vi "GetAttributeViInt32_SA-Gating_Sweep.vi"(8 "error in (no error)":errorcluster {"code" format="%.0x"}, 9 "AttributeID":u32(ring)=1150537 items=["SA_GATING_DELAY_COMPENSATION"=1150537, "SA_GATING_METHOD"=1150529, "SA_GATING_SOURCE"=1150531, "SA_GATING_TYPE"=1150532, "SA_LISTSWEEP_ATTENUATION_ELECTRONIC_POINTS"=1150655, "SA_LISTSWEEP_ATTENUATION_MECHANICAL_POINTS"=1150656, "SA_LISTSWEEP_BANDWIDTH_RESOLUTION_POINTS"=1150634, "SA_LISTSWEEP_BANDWIDTH_RESOLUTION_TYPE_POINTS"=1150635, "SA_LISTSWEEP_BANDWIDTH_VIDEO_POINTS"=1150636, "SA_LISTSWEEP_DETECTOR_POINTS"=1150653, "SA_LISTSWEEP_FREQUENCY_POINTS"=1150638, "SA_LISTSWEEP_FREQUENCY_SYNTHESIS"=1150639, "SA_LISTSWEEP_SEQUENCE_POINTS"=1150643, "SA_LISTSWEEP_TIME_POINTS"=1150651, "SA_LISTSWEEP_TRIGGER_DELAY_POINTS"=1150645, "SA_LISTSWEEP_TRIGGER_HOLDOFF_POINTS"=1150646, "SA_LISTSWEEP_TRIGGER_LEVEL_POINTS"=1150647, "SA_LISTSWEEP_TRIGGER_SLOPE"=1150657, "SA_LISTSWEEP_TRIGGER_SLOPE_POINTS"=1150648, "SA_LISTSWEEP_TRIGGER_SOURCE_POINTS"=1150649, "SA_LISTSWEEP_TRIGGER_SOURCE"=1150658, "SA_SWEEPCOUPLING_BANDWIDTH_SHAPE"=1150730, "SA_SWEEPCOUPLING_BANDWIDTH_TYPE"=1150731, "SA_SWEEPCOUPLING_SWEEP_POINTS"=1150724, "SA_SWEEPCOUPLING_SWEEP_TIME_AUTO_RULES"=1150732, "SA_SWEEPCOUPLING_SWEEP_TYPE_AUTO_RULES"=1150728, "SA_SWEEPCOUPLING_SWEEP_TYPE"=1150734], 11 "instrument handle":refnum<k15>) -> (0 "error out":errorcluster {"code" format="%.0x"}, 2 "AttributeValue":i32, 3 "instrument handle out":refnum<k15>)   [LabVIEW 2009, in "Keysight XSAn.lvlib"]
doc: "Gets an Int32 attribute from the instrument driver.\nThe following Attributes are supported:\n\nSA_GATING_DELAY_COMPENSATION\nSA_GATING_METHOD\nSA_GATING_SOURCE\nSA_GATING_TYPE\nSA_LISTSWEEP_ATTENUATION_ELECTRONIC_POINTS\nSA_LISTSWEEP_ATTENUATION_MECHANICAL_POINTS\nSA_LISTSWEEP_BANDWIDTH_RESOLUTION_POINTS\nSA_LISTSWEEP_BANDWIDTH_RESOLUTION_TYPE_POINTS\nSA_LISTSWEEP_BANDWIDTH_VIDEO_POINTS\nSA_LISTSWEEP_DETECTOR_POINTS\nSA_LISTSWEEP_FREQUENCY_POINTS\nSA_LISTSWEEP_FREQUENCY_SYNTHESIS\nSA_LISTSWEEP_SEQUENCE_POINTS\nSA_LISTSWEEP_TIME_POINTS\nSA_LISTSWEEP_TRIGGER_DELAY_POINTS\nSA_LISTSWEEP_TRIGGER_HOLDOFF_POINTS\nSA_LISTSWEEP_TRIGGER_LEVEL_POINTS\nSA_LISTSWEEP_TRIGGER_SLOPE\nSA_LISTSWEEP_TRIGGER_SLOPE_POINTS\nSA_LISTSWEEP_TRIGGER_SOURCE_POINTS\nSA_LISTSWEEP_TRIGGER_SOURCE\nSA_SWEEPCOUPLING_BANDWIDTH_SHAPE\nSA_SWEEPCOUPLING_BANDWIDTH_TYPE\nSA_SWEEPCOUPLING_SWEEP_POINTS\nSA_SWEEPCOUPLING_SWEEP_TIME_AUTO_RULES\nSA_SWEEPCOUPLING_SWEEP_TYPE_AUTO_RULES\nSA_SWEEPCOUPLING_SWEEP_TYPE"
uses:
  <instrlib>/Keysight XSAn/Keysight XSAn.lvlib
  AgXSAn.dll
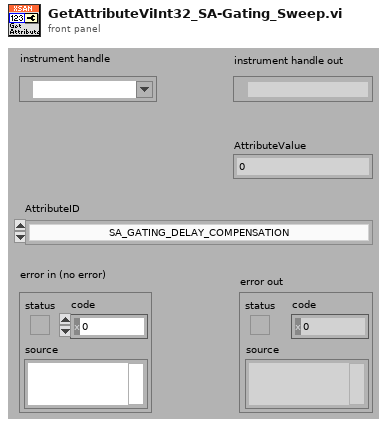
[diagram p1: front panel]
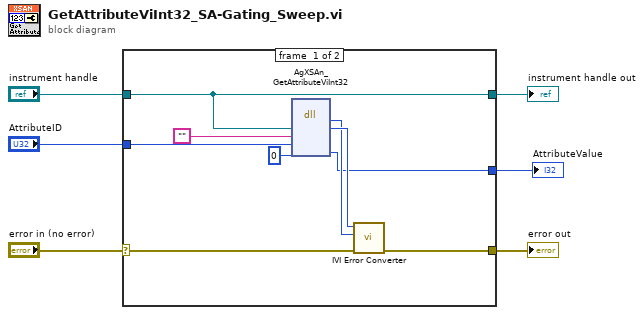
[diagram p0: block diagram]
diagram:
  n1 = case shown="No Error" "error in (no error)" {
    selector: "error in (no error)" -> [w13 w17]
    tunnel: [w12 w17] -> w6
    tunnel: "instrument handle" -> [w8 w16]
    tunnel: "AttributeID" -> [w11 _]
    tunnel: [w9 _] -> w2
    tunnel: [w8 w16] -> w1
    frame #0 {
      n2 = dll-call lib="AgXSAn**.dll" fn="AgXSAn_GetAttributeViInt32"("Vi"=w8, "RepCapIdentifier"="", "AttributeID"=w11, "AttributeValue"=0) -> ("return type"=w14:i32, "Vi"=w15:u32, "AttributeValue"=w9:i32)  [unwired: 5 in, 2 out]
      n3 = call <instrlib>:"IVI Error Converter.vi"("error in (no error)"=w13, "IVI error code (0)"=w14, "instrument handle"=w15) -> ("error out"=w12:errorcluster)  [unwired: 7 in, 1 out]
    }
    frame #1 {
    }
  }
  "error out" <- w6
  "instrument handle out" <- w1
  "AttributeValue" <- w2
